vi "Read Console Options.vi"(11 "Entry Console View Definition in":refnum<class "Entry Console View Definition.lvclass">) -> (3 "Entry Console View Definition out":refnum<class "Entry Console View Definition.lvclass">, 4 "Console Options":refnum<vi>[](array[refnum]))   [LabVIEW 2019, in "Entry Console View Definition.lvclass"]
uses:
  <vilib>/gpm_packages/@cs/Car-wash/Source/Entry Console View Definition/Entry Console View Definition/Entry Console View Definition.lvclass
  <vilib>/gpm_packages/@cs/Car-wash/Source/Entry Console View Definition/Entry Console View Definition/Entry Console View Definition.lvclass/Entry Console View Definition.ctl
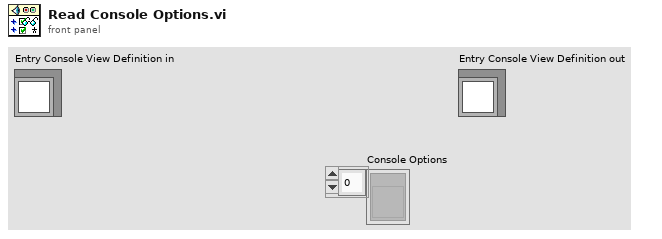
[diagram p1: front panel]
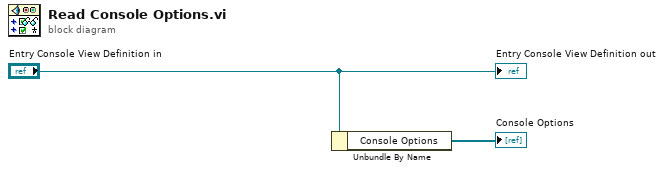
[diagram p0: block diagram]
diagram:
  n1 = Unbundle By Name("Entry Console View Definition in") -> ("Console Options"=→"Console Options":refnum<vi>[])
  "Entry Console View Definition out" <- "Entry Console View Definition in"
